vi "Draw Custom Scales.vi"(6 "Draw Area Size":cluster{"Width":u32, "Height":u32}={"Width"=400, "Height"=400}, 7 "Number of Points":cluster{"x":i32, "y":i32}, 8 "error in":errorcluster, 10 "Custom Graph Info":T1={"X Scale"={"X Scale Label"=TRUE, "X Scale Name"="Location", "X Scale Visible"=TRUE, "dx"=10.0}, "Y Scale"={"X Scale Label"=TRUE, "X Scale Name"="Time", "X Scale Visible"=TRUE, "dt"=4e-10}, "BackGround Color"=0}, 11 "picture in":picture) -> (0 "error out":errorcluster, 1 "Plot Area Size":cluster{"Width":u32, "Height":u32}, 2 "Offsets":cluster{"X offset":u32, "Y offset":u32}, 3 "picture out":picture)   [LabVIEW 2009]
doc: "Draws scales for a GPR graph, given the draw area size, number of points (for wiggle trace graphs) and a cluster describing scale and background info. This VI operates by setting all of the properties on a dummy graph, then getting an image of the dummy graph and drawing it on the picture."
uses:
  Controls/Display Info.ctl
panel:
  out "Template Graph":dbl[](graph)
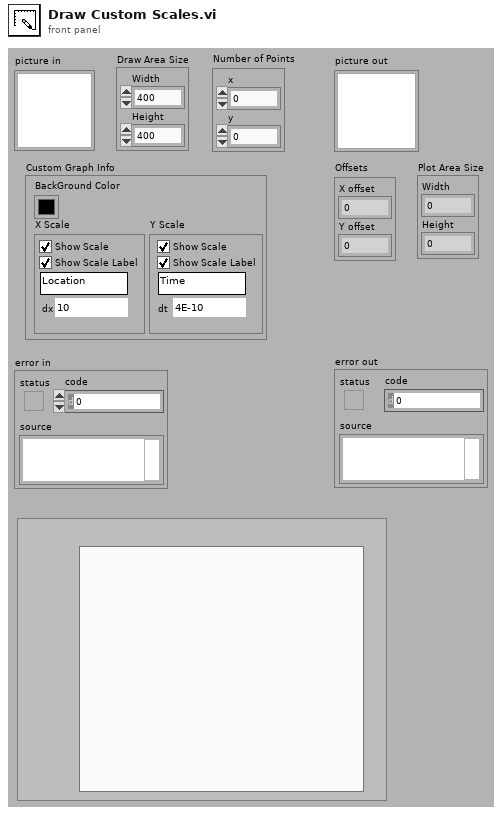
[diagram p1: front panel]
types:
  T1 = typedef "Display Info.ctl" = cluster{"X Scale":cluster{"X Scale Label":bool, "X Scale Name":string, "X Scale Visible":bool, "dx":dbl}, "Y Scale":cluster{"X Scale Label":bool, "X Scale Name":string, "X Scale Visible":bool, "dt":dbl}, "BackGround Color":u32}
  T2 = typedef "LVBoundsTypeDef.ctl" = cluster{"Width":u32, "Height":u32}
  T3 = typedef "LVRectTypeDef.ctl" = cluster{"left":i16, "top":i16, "right":i16, "bottom":i16}
  T4 = typedef "LVPositionTypeDef.ctl" = cluster{"Left":i32, "Top":i32}
  T5 = typedef "imagedata.ctl" = cluster{"image type":i32, "image depth":i32, "image":u8[], "mask":u8[], "colors":u32[], "Rectangle":cluster{"left":i16, "top":i16, "right":i16, "bottom":i16}}
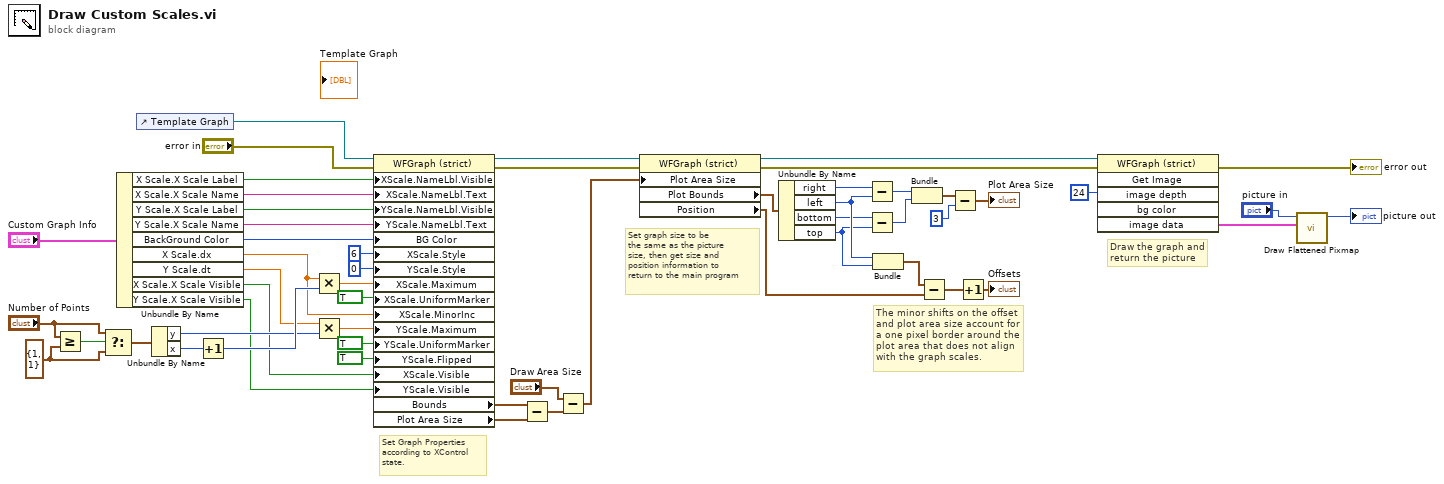
[diagram p0: block diagram]
diagram:
  w13 = cluster{"x":i32, "y":i32} {"x"=1, "y"=1} ("y")
  # "The minor shifts on the offset\nand plot area size account for\na one pixel border around the \nplot area that does not align \nwith the graph scales."
  # "Draw the graph and\nreturn the picture"
  # "Set graph size to be\nthe same as the picture\nsize, then get size and\nposition information to\nreturn to the main program"
  # "Set Graph Properties\naccording to XControl\nstate."
  n1 = Greater Or Equal?(x="Number of Points", y=w13) -> (x >= y?=w15:bool)
  n2 = Select(t="Number of Points", s=w15, f=w13) -> (s? t:f=w12:cluster{"x":i32, "y":i32})
  n3 = Unbundle By Name("Custom Graph Info") -> ("X Scale.X Scale Label"=w36:bool, "X Scale.X Scale Name"=w37:string, "Y Scale.X Scale Label"=w35:bool, "Y Scale.X Scale Name"=w34:string, "BackGround Color"=w26:u32, "X Scale.dx"=w23:dbl, "Y Scale.dt"=w22:dbl, "X Scale.X Scale Visible"=w4:bool, "Y Scale.X Scale Visible"=w5:bool)
  n4 = control-ref of="Template Graph"() -> (w11:refnum<vi>)
  n5 = Unbundle By Name(w12) -> ("y"=w47:i32, "x"=w49:i32)
  n6 = Increment(x=w49) -> (x+1=w48:i32)
  n7 = Multiply(x=w23, y=w48) -> (x*y=w25:dbl)
  n8 = Multiply(x=w22, y=w47) -> (x*y=w21:dbl)
  n9 = property on="Property Node" class="WFGraph (strict)"(reference=w11, error in="error in", "XScale.NameLbl.Visible"=w36, "XScale.NameLbl.Text"=w37, "YScale.NameLbl.Visible"=w35, "YScale.NameLbl.Text"=w34, "BG Color"=w26, "XScale.Style"=u8 6 ("X Scale.Style"), "YScale.Style"=u8 0 ("Y Scale.Style"), "XScale.Maximum"=w25, "XScale.UniformMarker"=TRUE ("X Scale.Uniform Marker Spacing?"), "XScale.MinorInc"=w23, "YScale.Maximum"=w21, "YScale.UniformMarker"=TRUE ("Y Scale.Uniform Marker Spacing?"), "YScale.Flipped"=TRUE ("Y Scale.Flipped"), "XScale.Visible"=w4, "YScale.Visible"=w5) -> (reference out=w46:refnum<vi>, error out=w44:errorcluster, "Bounds"=w9:T2, "Plot Area Size"=w8:T2)
  n10 = Subtract(x=w9, y=w8) -> (x-y=w7:T2)
  n11 = Subtract(x="Draw Area Size", y=w7) -> (x-y=w6:T2)
  n12 = property on="Property Node" class="WFGraph (strict)"(reference=w46, error in=w44, "Plot Area Size"=w6) -> (reference out=w18:refnum<vi>, error out=w17:errorcluster, "Plot Bounds"=w41:T3, "Position"=w40:T4)
  n13 = Unbundle By Name(w41) -> ("right"=w33:i16, "left"=w32:i16, "bottom"=w31:i16, "top"=w30:i16)
  n14 = Subtract(x=w33, y=w32) -> (x-y=w29:i16)
  n15 = Subtract(x=w31, y=w30) -> (x-y=w28:i16)
  n16 = Bundle("left"=w32, "top"=w30) -> (w45:cluster{"left":i16, "top":i16})  [unwired: 1 in]
  n17 = Bundle(w29, w28) -> (w3:cluster{i16, i16})  [unwired: 1 in]
  n18 = Subtract(x=w45, y=w40) -> (x-y=w43:T4)
  n19 = Subtract(x=w3, y=3 ("Image Depth")) -> (x-y=→"Plot Area Size":cluster{i32, i32})
  n20 = Increment(x=w43) -> (x+1=→"Offsets":T4)
  n21 = invoke class="WFGraph (strict)" method="Get Image"(reference=w18, error in=w17, "image depth"=24 ("Image Depth")) -> (error out=→"error out":errorcluster, "image data"=w52:T5)  [unwired: 3 in, 4 out]
  n22 = call <vilib>:"Draw Flattened Pixmap.vi"("image data"=w52, "picture"="picture in") -> ("new picture"=→"picture out":picture)  [unwired: 7 in]
